vi "初始化队列.vi"(8 "error in (no error)":errorcluster) -> (0 "error out":errorcluster, 2 "Queue Out":T1)   [LabVIEW 2015]
uses:
  Global/SeverGlobal.vi
panel:
  in  "Queue":T1
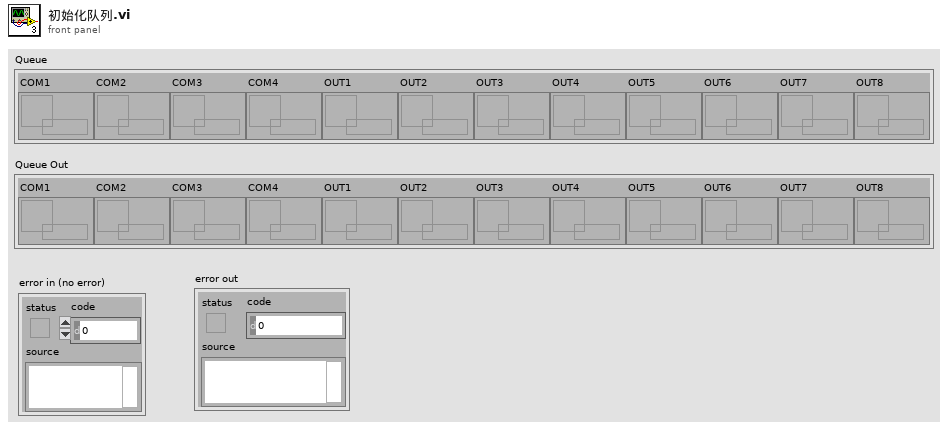
[diagram p1: front panel]
types:
  T1 = typedef "队列.ctl" = cluster{"COM1":refnum<queue>, "COM2":refnum<queue>, "COM3":refnum<queue>, "COM4":refnum<queue>, "OUT1":refnum<queue>, "OUT2":refnum<queue>, "OUT3":refnum<queue>, "OUT4":refnum<queue>, "OUT5":refnum<queue>, "OUT6":refnum<queue>, "OUT7":refnum<queue>, "OUT8":refnum<queue>}
  T2 = cluster{"TCP Ref":refnum<k5>, "IP":string, "userName":string, "A":u16, "COM":u16, "time":u32}
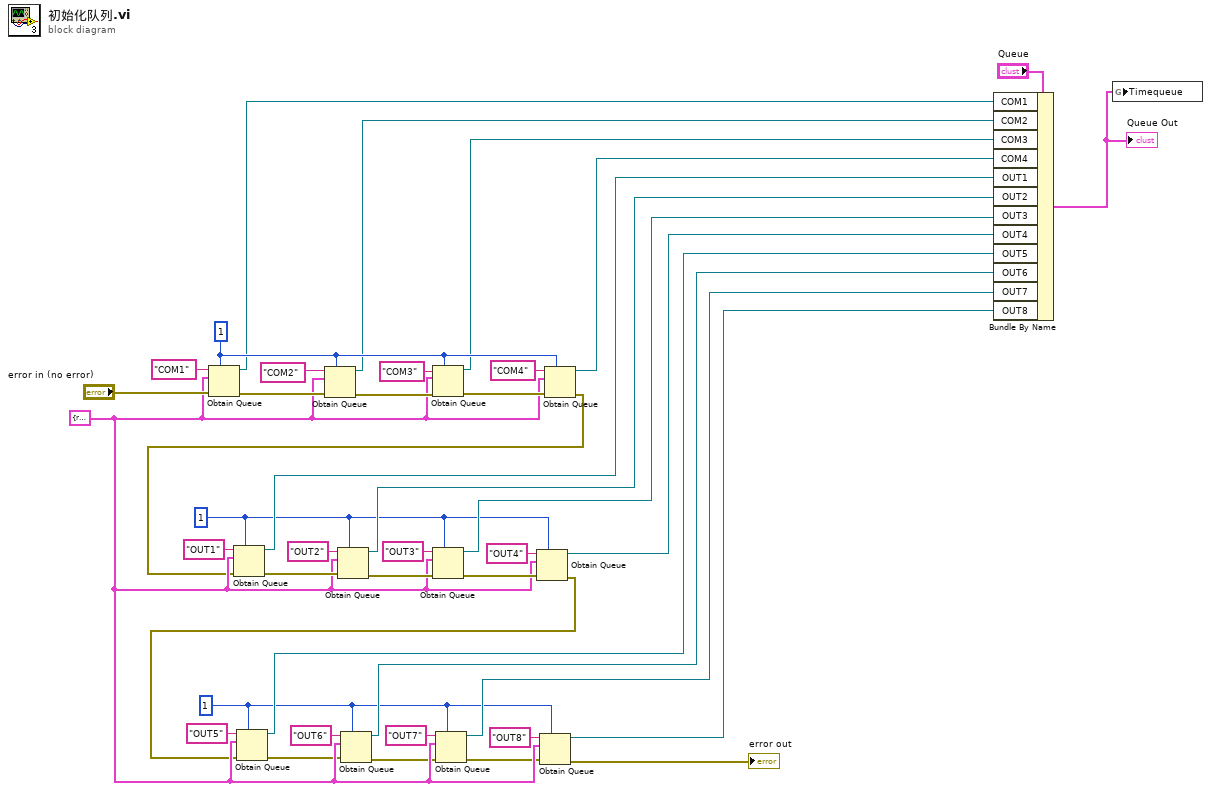
[diagram p0: block diagram]
diagram:
  w6 = 1 ("max queue size (-1, unlimited)")
  w7 = 1 ("max queue size (-1, unlimited)")
  w38 = 1 ("max queue size (-1, unlimited)")
  w17 = T2 {"TCP Ref"=refnum, "IP"="", "userName"="", "A"=0, "COM"=0, "time"=0} ("RF_Now")
  n1 = Obtain Queue(max queue size (-1, unlimited)=w38, name (unnamed)="COM1", element data type=w17, error in (no error)="error in (no error)") -> (queue out=w33:refnum<queue>, error out=w41:errorcluster)  [unwired: 1 in, 1 out]
  n2 = Obtain Queue(max queue size (-1, unlimited)=w38, name (unnamed)="COM2", element data type=w17, error in (no error)=w41) -> (queue out=w32:refnum<queue>, error out=w39:errorcluster)  [unwired: 1 in, 1 out]
  n3 = Obtain Queue(max queue size (-1, unlimited)=w38, name (unnamed)="COM3", element data type=w17, error in (no error)=w39) -> (queue out=w31:refnum<queue>, error out=w40:errorcluster)  [unwired: 1 in, 1 out]
  n4 = Obtain Queue(max queue size (-1, unlimited)=w38, name (unnamed)="COM4", element data type=w17, error in (no error)=w40) -> (queue out=w30:refnum<queue>, error out=w2:errorcluster)  [unwired: 1 in, 1 out]
  n5 = Obtain Queue(max queue size (-1, unlimited)=w7, name (unnamed)="OUT1", element data type=w17, error in (no error)=w2) -> (queue out=w16:refnum<queue>, error out=w20:errorcluster)  [unwired: 1 in, 1 out]
  n6 = Obtain Queue(max queue size (-1, unlimited)=w7, name (unnamed)="OUT2", element data type=w17, error in (no error)=w20) -> (queue out=w15:refnum<queue>, error out=w19:errorcluster)  [unwired: 1 in, 1 out]
  n7 = Obtain Queue(max queue size (-1, unlimited)=w7, name (unnamed)="OUT3", element data type=w17, error in (no error)=w19) -> (queue out=w14:refnum<queue>, error out=w18:errorcluster)  [unwired: 1 in, 1 out]
  n8 = Obtain Queue(max queue size (-1, unlimited)=w7, name (unnamed)="OUT4", element data type=w17, error in (no error)=w18) -> (queue out=w13:refnum<queue>, error out=w1:errorcluster)  [unwired: 1 in, 1 out]
  n9 = Obtain Queue(max queue size (-1, unlimited)=w6, name (unnamed)="OUT5", element data type=w17, error in (no error)=w1) -> (queue out=w12:refnum<queue>, error out=w5:errorcluster)  [unwired: 1 in, 1 out]
  n10 = Obtain Queue(max queue size (-1, unlimited)=w6, name (unnamed)="OUT6", element data type=w17, error in (no error)=w5) -> (queue out=w11:refnum<queue>, error out=w4:errorcluster)  [unwired: 1 in, 1 out]
  n11 = Obtain Queue(max queue size (-1, unlimited)=w6, name (unnamed)="OUT7", element data type=w17, error in (no error)=w4) -> (queue out=w10:refnum<queue>, error out=w3:errorcluster)  [unwired: 1 in, 1 out]
  n12 = Obtain Queue(max queue size (-1, unlimited)=w6, name (unnamed)="OUT8", element data type=w17, error in (no error)=w3) -> (queue out=w9:refnum<queue>, error out=→"error out":errorcluster)  [unwired: 1 in, 1 out]
  n13 = Bundle By Name(cluster="Queue", "COM1"=w33, "COM2"=w32, "COM3"=w31, "COM4"=w30, "OUT1"=w16, "OUT2"=w15, "OUT3"=w14, "OUT4"=w13, "OUT5"=w12, "OUT6"=w11, "OUT7"=w10, "OUT8"=w9) -> (w29:T1)
  "Queue Out" <- w29
  n14 = global write "SeverGlobal.vi" "Timequeue"(w29) -> ()
